vi "get_filename_from_timestamp.vi"(10 "Suffix":string, 11 "Path":path) -> (1 "Log":path, 2 "Tif":path, 3 "Bin":path)   [LabVIEW 2016]
doc: "Produces useful filenames (paths) by adding a suffic and a filetype to a path."
panel:
  in  "Record Path":path
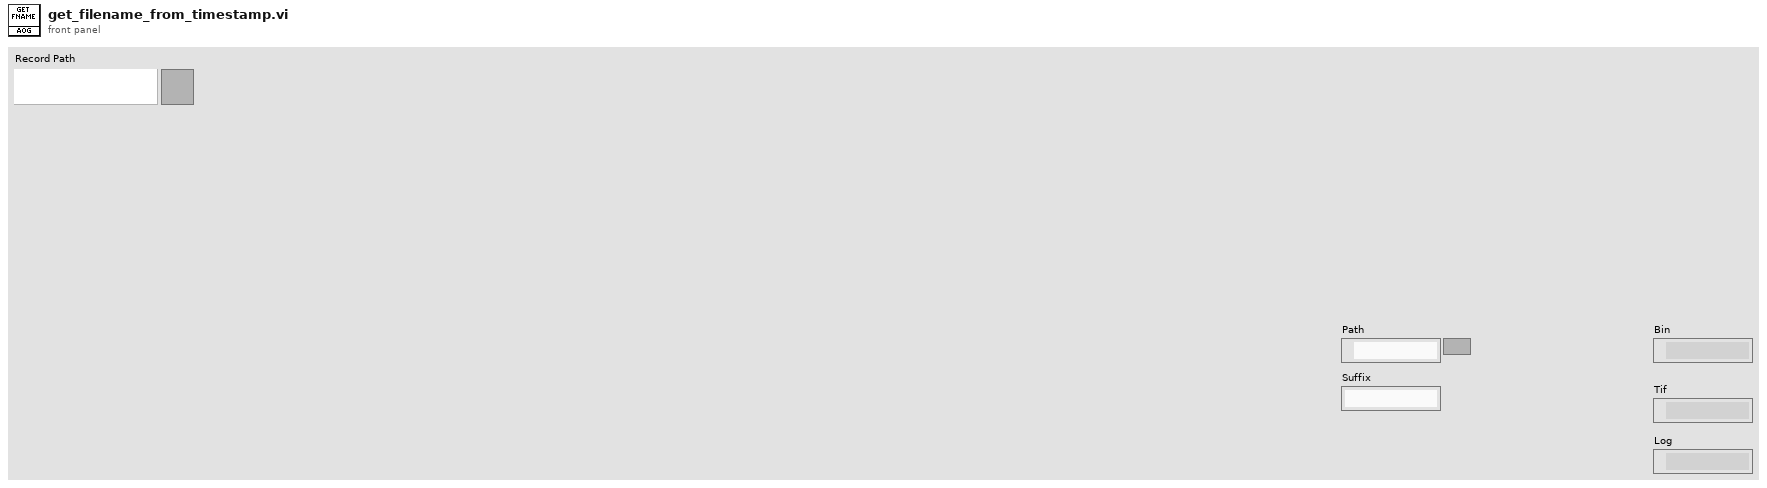
[diagram p1: front panel]
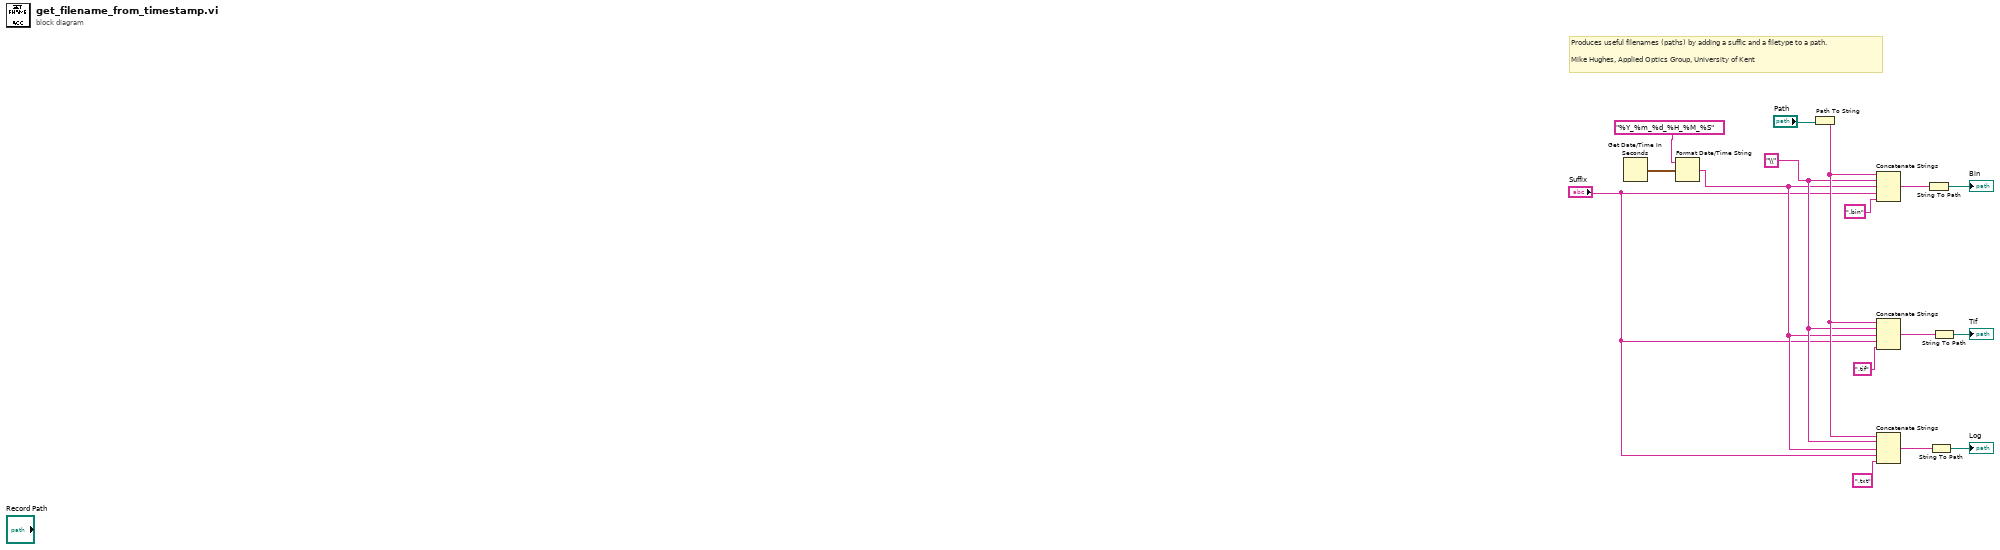
[diagram p0: block diagram]
diagram:
  w8 = "\\"
  # "Produces useful filenames (paths) by adding a suffic and a filetype to a path.\n\nMike Hughes, Applied Optics Group, University of Kent"
  n1 = Get Date/Time In Seconds() -> (seconds since 1Jan1904=w16:timestamp)
  n2 = Format Date/Time String(time format string (%c)="%Y_%m_%d_%H_%M_%S", seconds (now)=w16) -> (date/time string=w7:string)  [unwired: 1 in]
  n3 = Path To String(path="Path") -> (string=w9:string)
  n4 = Concatenate Strings(w9, w8, w7, "Suffix", ".bin") -> (w14:string)
  n5 = Concatenate Strings(w9, w8, w7, "Suffix", ".tif") -> (w11:string)
  n6 = Concatenate Strings(w9, w8, w7, "Suffix", ".txt") -> (w6:string)
  n7 = String To Path(string=w14) -> (path=→"Bin":path)
  n8 = String To Path(string=w6) -> (path=→"Log":path)
  n9 = String To Path(string=w11) -> (path=→"Tif":path)
